vi "HIOKI PW3390 Conf CH A Frequency.vi"(0 "VISA Resource":refnum<visa-resource-name>, 1 "Set/Query (F: Set)":bool, 5 "Unit (3: Nm)":enum16{"V", "Hz", "mNm", "Nm", "kNm"}(ring)=enum."Nm", 7 "Torq (1)":i32=1 min=1 max=999, 9 "Range (60k, 30k)":cluster{"fc":i32, "fd":i32}={"fc"=60000, "fd"=30000} {"fd" min=1000 max=48000 step=1000; "fc" min=3000 max=98000 step=1000}, 11 "error in (no error)":errorcluster, 12 "OPC query (T: ON)":bool=TRUE, 13 "Error Out (F: Off)":bool) -> (3 "CH A input out":enum16{"FREQ", "DC"}(ring), 4 "VISA Resource out":refnum<visa-resource-name>, 6 "Unit out":enum16{"V", "Hz", "mNm", "Nm", "kNm"}(ring)=enum."Nm", 8 "Torq out":i32=1, 10 "Range out":cluster{"fc":i32, "fd":i32}={"fc"=60000, "fd"=30000}, 15 "error out":errorcluster)   [LabVIEW 2009]
doc: "Sets and reads the functions related to the Motor Analysis Option's Channel A input frequency.\n\nSet/Query\n Set: Send the setting commands for the device.\n Query: Query the setting of the device.\n\nUnit\n Sets the Channel A unit.\n\nTorq\n Sets the torque value of Channel A.\n Input Range: 1 - 999\n\nRange\n Sets the Channel A's frequency ranges fc and fd.\n Input Range fc: 3000 - 98000\n Intput Range fd: 1000 - 48000\n<B>Note</B>\nCan be set when it is fc + fd < 100kHz and fc - fd > 1kHz.\nAlways set fc and fd in multiples of 1000."
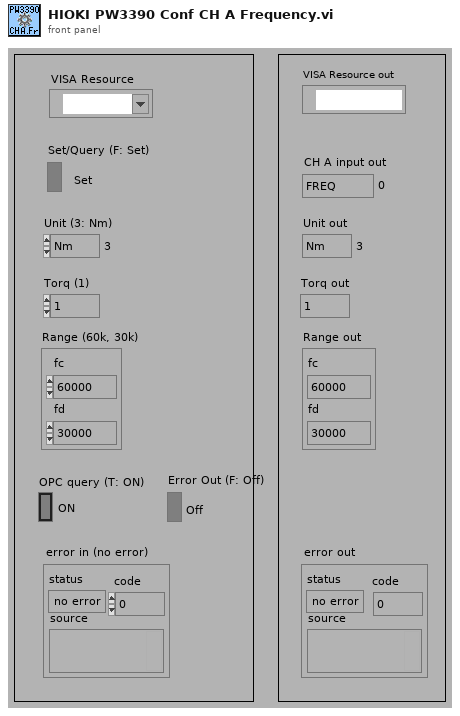
[diagram p1: front panel]
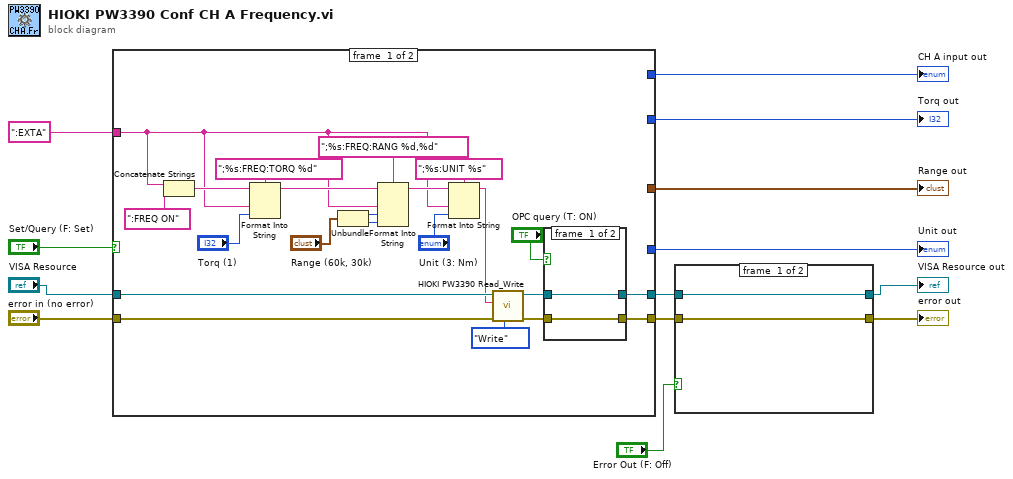
[diagram p0: block diagram]
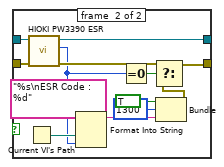
[diagram p2: hidden frame]
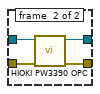
[diagram p3: hidden frame]
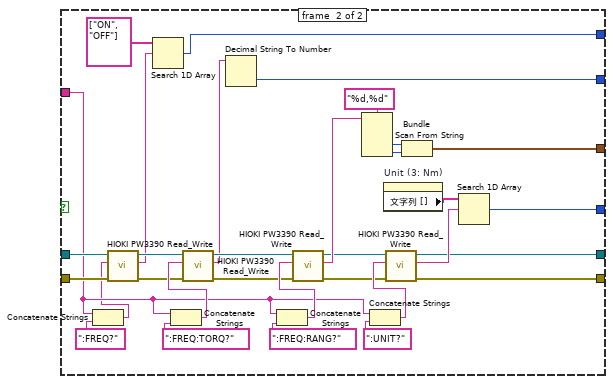
[diagram p4: hidden frame]
diagram:
  n1 = case shown="FALSE" "Set/Query (F: Set)" {
    tunnel: "error in (no error)" -> [w31 w48]
    tunnel: [w18 w61] -> w6
    tunnel: "VISA Resource" -> [w32 w51]
    tunnel: [w19 w62] -> w5
    tunnel: [_ w60] -> w11
    tunnel: ":EXTA" -> [w15 w47]
    tunnel: [_ w54] -> w10
    tunnel: [_ w70] -> w9
    tunnel: [_ w42] -> w1
    frame #0 {
      n2 = Concatenate Strings(w15, ":FREQ ON") -> (w16:string)
      n3 = Format Into String(format string=";%s:FREQ:TORQ %d", initial string=w16, w15, "Torq (1)") -> (resulting string=w24:string)  [unwired: 1 in, 1 out]
      n4 = Unbundle("Range (60k, 30k)") -> ("fc"=w27:i32, "fd"=w26:i32)
      n5 = Format Into String(format string=";%s:FREQ:RANG %d,%d", initial string=w24, w15, w27, w26) -> (resulting string=w17:string)  [unwired: 1 in, 1 out]
      n6 = Format Into String(format string=";%s:UNIT %s", initial string=w17, w15, "Unit (3: Nm)") -> (resulting string=w23:string)  [unwired: 1 in, 1 out]
      n7 = call <instrlib>:"HIOKI PW3390 Read_Write.vi"("Read/Write"=enum16{"Read", "Write"}."Write", "error in (no error)"=w31, "data in"=w23, "VISA Resource"=w32) -> ("error out"=w20:errorcluster, "VISA Resource out"=w21:refnum<visa-resource-name>)  [unwired: 5 in, 1 out]
      n8 = case shown="TRUE" "OPC query (T: ON)" {
        tunnel: [w37 w41] -> w19
        tunnel: [w36 w40] -> w18
        tunnel: w21 -> [w37 w39]
        tunnel: w20 -> [w36 w38]
        frame #0 {
        }
        frame #1 {
          n9 = call <instrlib>:"HIOKI PW3390 OPC.vi"("error in (no error)"=w38, "VISA Resource"=w39) -> ("error out"=w40:errorcluster, "VISA Resource out"=w41:refnum<visa-resource-name>)  [unwired: 7 in, 1 out]
        }
      }
    }
    frame #1 {
      n10 = Concatenate Strings(w47, ":FREQ?" ("文字列")) -> (w45:string)
      n11 = call <instrlib>:"HIOKI PW3390 Read_Write.vi"("error in (no error)"=w48, "data in"=w45, "VISA Resource"=w51) -> ("error out"=w49:errorcluster, "data out"=w43:string, "VISA Resource out"=w50:refnum<visa-resource-name>)  [unwired: 6 in]
      n12 = Search 1D Array(1D array=string[] ["ON", "OFF"] ("文字列配列"), element=w43) -> (index of element=w42:i32)  [unwired: 1 in]
      n13 = Concatenate Strings(w47, ":FREQ:TORQ?") -> (w65:string)
      n14 = call <instrlib>:"HIOKI PW3390 Read_Write.vi"("error in (no error)"=w49, "data in"=w65, "VISA Resource"=w50) -> ("error out"=w67:errorcluster, "data out"=w59:string, "VISA Resource out"=w68:refnum<visa-resource-name>)  [unwired: 6 in]
      n15 = Decimal String To Number(string=w59) -> (number=w60:i32)  [unwired: 2 in, 1 out]
      n16 = Concatenate Strings(w47, ":FREQ:RANG?") -> (w69:string)
      n17 = call <instrlib>:"HIOKI PW3390 Read_Write.vi"("error in (no error)"=w67, "data in"=w69, "VISA Resource"=w68) -> ("error out"=w52:errorcluster, "data out"=w58:string, "VISA Resource out"=w53:refnum<visa-resource-name>)  [unwired: 6 in]
      n18 = Scan From String(format string="%d,%d" ("形式文字列"), input string=w58) -> (output 1=w56:i32, output 2=w55:i32)  [unwired: 4 in, 3 out]
      n19 = Concatenate Strings(w47, ":UNIT?") -> (w66:string)
      n20 = property on="Unit (3: Nm)" class="Enum (strict)"() -> ("文字列 []"=w64:string[])  [unwired: 2 in, 2 out]
      n21 = call <instrlib>:"HIOKI PW3390 Read_Write.vi"("error in (no error)"=w52, "data in"=w66, "VISA Resource"=w53) -> ("error out"=w61:errorcluster, "data out"=w63:string, "VISA Resource out"=w62:refnum<visa-resource-name>)  [unwired: 6 in]
      n22 = Bundle(w56, w55) -> (w54:cluster{i32, i32})  [unwired: 1 in]
      n23 = Search 1D Array(1D array=w64, element=w63) -> (index of element=w70:i32)  [unwired: 1 in]
    }
  }
  "Torq out" <- w11
  "Unit out" <- w9
  "Range out" <- w10
  "CH A input out" <- w1
  n24 = case shown="TRUE" "Error Out (F: Off)" {
    tunnel: w5 -> [w75 w88]
    tunnel: w6 -> [w74 w87]
    tunnel: [w74 w77] -> w4
    tunnel: [w75 w86] -> w2
    frame #0 {
    }
    frame #1 {
      n25 = Current VI's Path() -> (path=w84:path)
      n26 = call <instrlib>:"HIOKI PW3390 ESR.vi"("error in (no error)"=w87, "VISA Resource"=w88) -> ("error out"=w78:errorcluster, "Output Value"=w76:u8, "VISA Resource out"=w86:refnum<visa-resource-name>)  [unwired: 6 in, 1 out]
      n27 = Format Into String(format string="%s\nESR Code : %d", w84, w76) -> (resulting string=w80:string)  [unwired: 2 in, 1 out]
      n28 = Equal To 0?(x=w76) -> (x = 0?=w85:bool)
      n29 = Bundle("status"=TRUE, "code"=1300, w80) -> (w79:cluster{"status":bool, "code":i32, string})  [unwired: 1 in]
      n30 = Select(t=w78, s=w85, f=w79) -> (s? t:f=w77:errorcluster)
    }
  }
  "error out" <- w4
  "VISA Resource out" <- w2
